vi "String to Array.vi"(7 "Quoted Strings? (F)":bool, 11 "Array String In":string) -> (3 "JSON Strings":string[](array[string]))   [LabVIEW 2020, in "JSON.lvlib"]
uses:
  JSON.lvlib
  JSON Item Type.ctl
panel:
  out "Types":T1[](array[typedef])
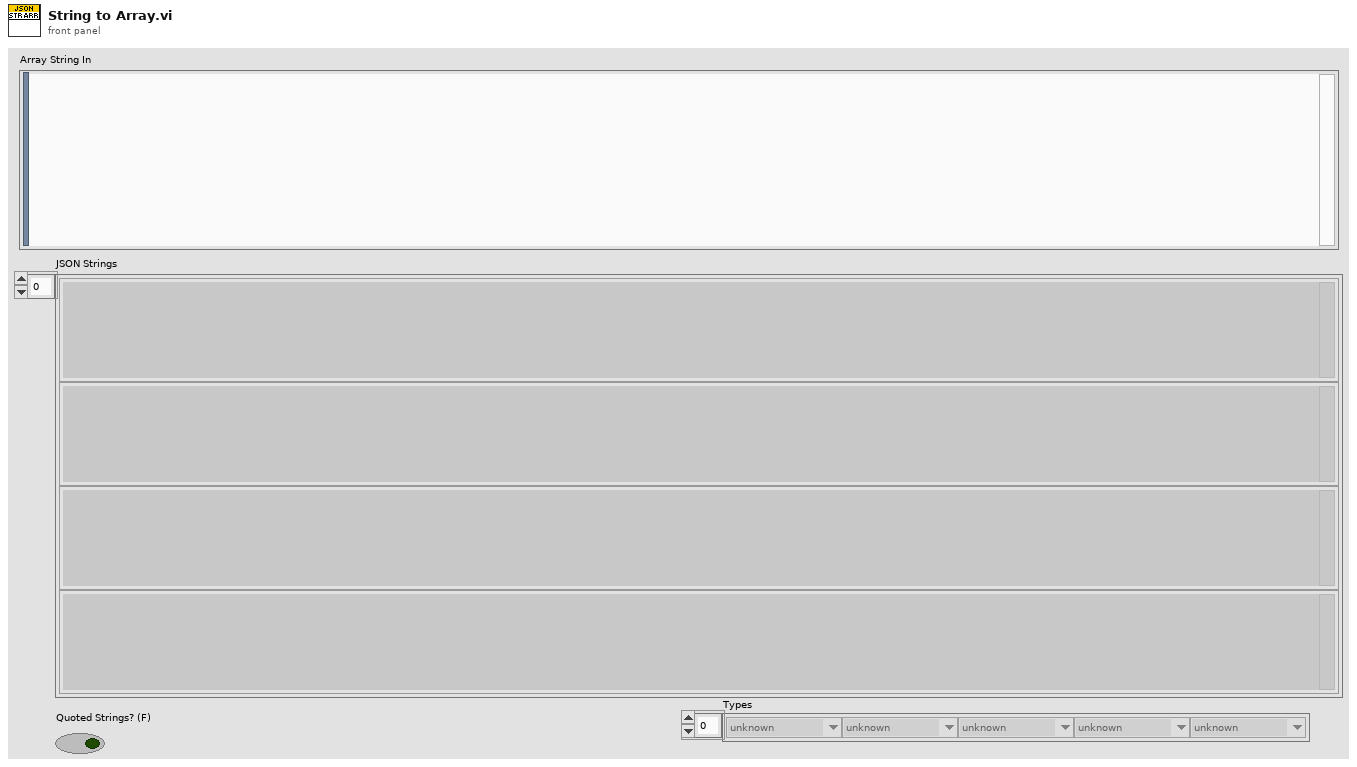
[diagram p1: front panel]
types:
  T1 = typedef "JSON.lvlib/JSON Item Type.ctl" = enum16{"unknown", "null", "Array", "Object", "String", "Number", "Boolean"}
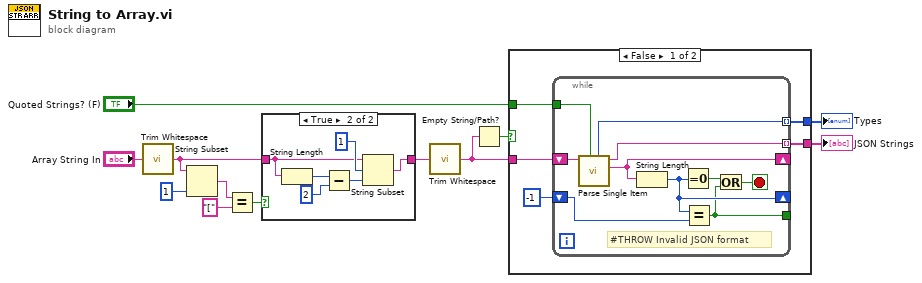
[diagram p0: block diagram]
diagram:
  n1 = call <vilib>:"Trim Whitespace.vi"("string"="Array String In") -> ("trimmed string"=w5:string)  [unwired: 1 in]
  n2 = String Subset(string=w5, length (rest)=1 ("length (rest)")) -> (substring=w8:string)  [unwired: 1 in]
  n3 = Equal?(x=w8, y="[") -> (x = y?=w6:bool)
  n4 = case shown="True" w6 {
    tunnel: w5 -> [w13 w18]
    tunnel: [w13 w14] -> w3
    frame False {
    }
    frame True {
      n5 = String Length(string=w18) -> (length=w17:i32)
      n6 = Subtract(x=w17, y=2) -> (x-y=w15:i32)
      n7 = String Subset(string=w18, offset (0)=1, length (rest)=w15) -> (substring=w14:string)
    }
  }
  n8 = call <vilib>:"Trim Whitespace.vi"("string"=w3) -> ("trimmed string"=w1:string)  [unwired: 1 in]
  n9 = Empty String/Path?(string/path=w1) -> (empty?=w4:bool)
  n10 = case shown="False" w4 {
    tunnel: [w24 _] -> w12
    tunnel: [w23 _] -> w11
    tunnel: w1 -> [w22 _]
    tunnel: "Quoted Strings? (F)" -> [w20 _]
    frame False {
      n11 = while {
        shift-right: [w25] -> _
        shift-left: w22 -> [w28]
        tunnel: [w27] -> w24 mode=indexing
        tunnel: [w26] -> w23 mode=indexing
        shift-right: [w32] -> _
        shift-left: -1 -> [w33]
        tunnel: [w30] -> _
        tunnel: w20 -> [w29]
        stop <- w31 stop-if-true
        # "#THROW Invalid JSON format"
        n12 = call "Parse Single Item.vi"("Quoted String? (F)"=w29, "String In"=w28) -> ("Remaining"=w25:string, "Item"=w27:string, "JSON Item Type"=w26:T1)  [unwired: 7 in]
        n13 = String Length(string=w25) -> (length=w32:i32)
        n14 = Equal To 0?(x=w32) -> (x = 0?=w34:bool)
        n15 = Equal?(x=w32, y=w33) -> (x = y?=w30:bool)
        n16 = Or(x=w34, y=w30) -> (x .or. y?=w31:bool)
      }
    }
    frame True {
    }
  }
  "JSON Strings" <- w12
  "Types" <- w11
